vi "Get Actor Events.vi"(8 "error in (no error)":errorcluster, 10 "Request Timeout":i32=-1, 11 "Message Enqueuer in":refnum<class "Message Enqueuer.lvclass">) -> (0 "error out":errorcluster, 1 "timed out?":bool, 2 "Actor Events":T1, 3 "Message Enqueuer out":refnum<class "Message Enqueuer.lvclass">)   [LabVIEW 2017, in "Command Handler.lvlib" / "Return Events Msg.lvclass"]
uses:
  Return Events Msg.lvclass
  <vilib>/ActorFramework/Message Enqueuer/Message Enqueuer.lvclass
  Command Handler/Type Defs/Event Cluster.ctl
  Command Parent/Command.lvclass
  Command Handler/Type Defs/Command Handler Data.ctl
  Return Events Msg.lvclass/Return Events Msg.ctl
  <vilib>/ActorFramework/Message Enqueuer/Message Enqueuer.lvclass/Message Enqueuer.ctl
  <vilib>/ActorFramework/Message Enqueuer/Enqueue.vi
  C:/Program Files (x86)/National Instruments/LabVIEW 2017/vi.lib/ActorFramework/Message/Message.lvclass
  <vilib>/ActorFramework/Message Priority Queue/Priority Enqueue.vi
  Command Handler/Command Handler.lvclass
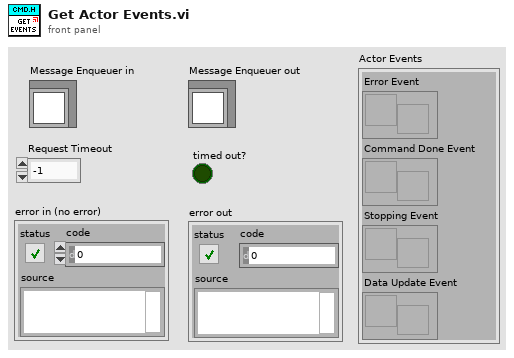
[diagram p1: front panel]
types:
  T1 = typedef "Command Handler.lvlib/Command Handler.lvclass/Event Cluster.ctl" = cluster{"Error Event":refnum<user-event>, "Command Done Event":refnum<user-event>, "Stopping Event":refnum<user-event>, "Data Update Event":refnum<user-event>}
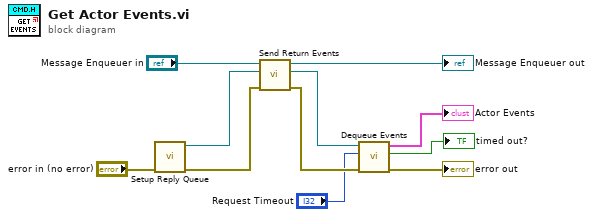
[diagram p0: block diagram]
diagram:
  n1 = call "Setup Reply Queue.vi"("error in (no error)"="error in (no error)") -> ("error out"=w7:errorcluster, "Queue out"=w10:refnum<queue>)  [unwired: 9 in]
  n2 = call "Send Return Events.vi"("error in (no error)"=w7, "Event Reply Queue In"=w10, "Message Enqueuer"="Message Enqueuer in") -> ("error out"=w8:errorcluster, "Event Reply Queue Out"=w5:refnum<queue>, "Message Enqueuer out"=→"Message Enqueuer out":refnum<class "Message Enqueuer.lvclass">)  [unwired: 6 in]
  n3 = call "Dequeue Events.vi"("error in (no error)"=w8, "timeout in ms (-1)"="Request Timeout", "Queue in"=w5) -> ("error out"=→"error out":errorcluster, "timed out?"=→"timed out?":bool, "Actor Events"=→"Actor Events":T1)  [unwired: 6 in]
